vi "Update Build Version.vi"(8 "error in (no error)":errorcluster, 11 "PostBuildSupport in":refnum<class "PostBuildSupport.lvclass">) -> (0 "error out":errorcluster, 3 "PostBuildSupport out":refnum<class "PostBuildSupport.lvclass">)   [LabVIEW 2016, in "build support.lvlib" / "PostBuildSupport.lvclass"]
uses:
  PostBuildSupport.lvclass
  <vilib>/AppBuilder/AB_API_Simple/Build Specification Version.ctl
  PostBuildSupport.lvclass/PostBuildSupport.ctl
  <vilib>/AppBuilder/AB_API_Simple/Set Build Specification Version (path).vi
  <vilib>/AppBuilder/AB_API_Simple/NI_App_Builder_API.lvlib
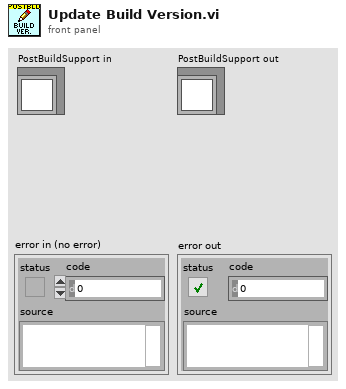
[diagram p1: front panel]
types:
  T1 = typedef "NI_App_Builder_API.lvlib/Build Specification Version.ctl" = cluster{"Major":u16, "Minor":u16, "Fix":u16, "Build":u16}
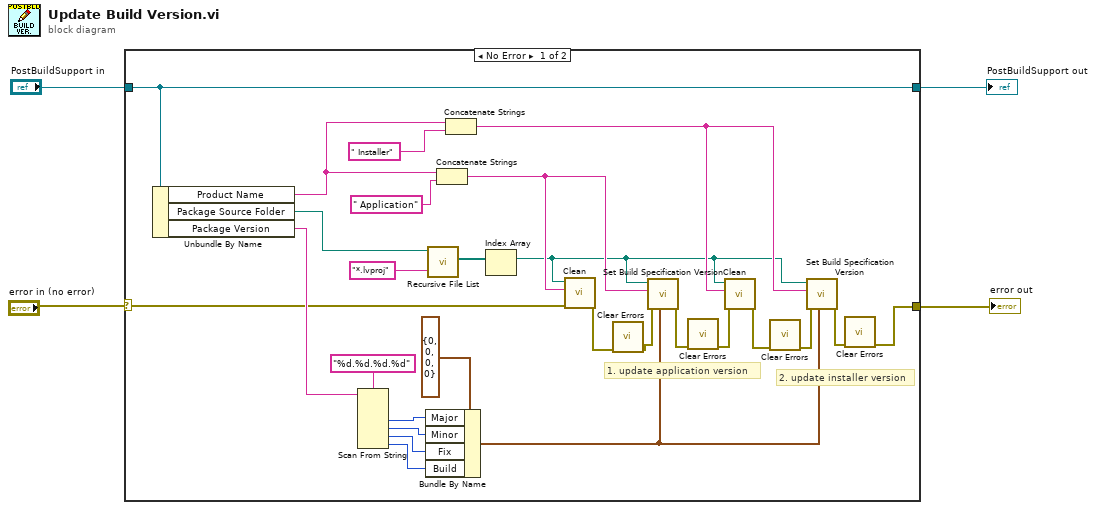
[diagram p0: block diagram]
diagram:
  n1 = case shown="No Error" "error in (no error)" {
    selector: "error in (no error)" -> [w13 w32]
    tunnel: [w5 w32] -> w4
    tunnel: "PostBuildSupport in" -> [w14 w33]
    tunnel: [w14 w33] -> w2
    frame No Error {
      # "2. update installer version"
      # "1. update application version"
      n2 = Unbundle By Name(w14) -> ("Product Name"=w16:string, "Package Source Folder"=w17:path, "Package Version"=w15:string)
      n3 = Scan From String(format string="%d.%d.%d.%d", input string=w15) -> (output 1=w27:i32, output 2=w30:i32, output 3=w26:i32, output 4=w29:i32)  [unwired: 6 in, 3 out]
      n4 = Bundle By Name(cluster=T1 {"Major"=0, "Minor"=0, "Fix"=0, "Build"=0} ("Build Specification Version"), "Major"=w27, "Minor"=w30, "Fix"=w26, "Build"=w29) -> (w31:T1)
      n5 = call <vilib>:"Recursive File List.vi"("pattern"="*.lvproj", "Folder Path"=w17) -> ("All Files in Dir"=w19:path[])  [unwired: 5 in, 4 out]
      n6 = Concatenate Strings(w16, " Application" ("Name of target (My Computer)")) -> (w23:string)
      n7 = Concatenate Strings(w16, " Installer" ("Name of target (My Computer)")) -> (w21:string)
      n8 = Index Array(array=w19) -> (element=w18:path)  [unwired: 1 in]
      n9 = call <vilib>:"Clean.vi"("error in (no error)"=w13, "Name of build specification (if empty: clean all)"=w23, "Path to project"=w18) -> ("error out"=w9:errorcluster)  [unwired: 8 in]
      n10 = call <vilib>:"Clear Errors.vi"("error in (no error)"=w9) -> ("error out"=w12:errorcluster)  [unwired: 5 in, 1 out]
      n11 = call-poly <vilib>:"Set Build Specification Version.vi"("Build Specification Version"=w31, "error in (no error)"=w12, "Name of build specification"=w23, "Path to project"=w18) -> ("error out"=w11:errorcluster)  [unwired: 7 in]
      n12 = call <vilib>:"Clear Errors.vi"("error in (no error)"=w11) -> ("error out"=w10:errorcluster)  [unwired: 5 in, 1 out]
      n13 = call <vilib>:"Clean.vi"("error in (no error)"=w10, "Name of build specification (if empty: clean all)"=w21, "Path to project"=w18) -> ("error out"=w8:errorcluster)  [unwired: 8 in]
      n14 = call <vilib>:"Clear Errors.vi"("error in (no error)"=w8) -> ("error out"=w7:errorcluster)  [unwired: 5 in, 1 out]
      n15 = call-poly <vilib>:"Set Build Specification Version.vi"("Build Specification Version"=w31, "error in (no error)"=w7, "Name of build specification"=w21, "Path to project"=w18) -> ("error out"=w6:errorcluster)  [unwired: 7 in]
      n16 = call <vilib>:"Clear Errors.vi"("error in (no error)"=w6) -> ("error out"=w5:errorcluster)  [unwired: 5 in, 1 out]
    }
    frame Error {
    }
  }
  "error out" <- w4
  "PostBuildSupport out" <- w2
